vi "Send Software Trigger Core.vi"(8 "error in (no error)":errorcluster, 11 "IVI_DMM in":refnum<class "IVI_DMM.lvclass">) -> (0 "error out":errorcluster, 3 "IVI_DMM out":refnum<class "IVI_DMM.lvclass">)   [LabVIEW 2015, in "IVI_DMM.lvlib" / "IVI_DMM.lvclass"]
doc: "This VI sends a command to trigger the DMM. Call this VI if you pass IVIDMM_VAL_SOFTWARE_TRIG for the Trigger Source parameter of the Configure Trigger VI or the Sample Trigger parameter of the Configure Multi-Point [MP] VI.\n\nNotes:\n\n(1) This VI is part of the IviDmmSoftwareTrigger [SWT] extension group.\n\n(2) If neither the IviDmm>Trigger>Trigger Source nor the IviDmm>Multi-Point Acquisition>Sample Trigger [MP] property is set to the IVIDMM_VAL_SOFTWARE_TRIG value, this VI returns an error.\n\n(3) This VI does not check the instrument status. Typically, you call this VI only in a sequence of calls to other low-level driver VIs. The sequence performs one operation. You use the low-level VIs to optimize one or more aspects of interaction with the instrument. If you want to check the instrument status, call the Error-Query VI at the conclusion of the sequence."
uses:
  IVI_DMM.lvclass
  IVI_DMM.lvclass/IVI_DMM.ctl
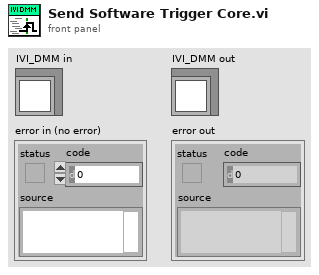
[diagram p1: front panel]
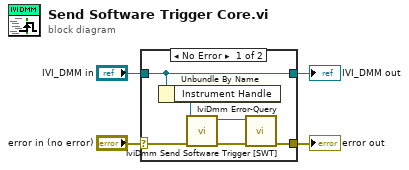
[diagram p0: block diagram]
diagram:
  n1 = case shown="No Error" "error in (no error)" {
    selector: "error in (no error)" -> [w8 w12]
    tunnel: [w5 w12] -> w3
    tunnel: [w10 w11] -> w1
    tunnel: "IVI_DMM in" -> [w10 w11]
    frame No Error {
      n2 = Unbundle By Name(w10) -> ("Instrument Handle"=w9:refnum<k15>)
      n3 = call <vilib>:"IviDmm Send Software Trigger [SWT].vi"("error in (no error)"=w8, "instrument handle"=w9) -> ("error out"=w6:errorcluster, "instrument handle out"=w7:refnum<k15>)  [unwired: 8 in]
      n4 = call <vilib>:"IviDmm Error-Query.vi"("error in (no error)"=w6, "instrument handle"=w7) -> ("error out"=w5:errorcluster)  [unwired: 6 in, 3 out]
    }
    frame Error {
    }
  }
  "error out" <- w3
  "IVI_DMM out" <- w1
